vi "Get Data Refs.vi"(8 "error in (no error)":errorcluster, 9 "Access":T3, 10 "References":T1[](array[typedef]) format="%.0x", 11 "Item Ref in":T1 format="%.0x") -> (0 "error out":errorcluster, 2 "Data References":T2[](array[typedef]) format="%.0x", 3 "Device Ref out":T1 format="%.0x")   [LabVIEW 2021]
uses:
  <vilib>/NI VeriStand/Custom Device API/Data Access Type.ctl
  <vilib>/NI VeriStand/Custom Device API/Custom Device Item Ref.ctl
  <vilib>/NI VeriStand/Custom Device API/Data Reference.ctl
  <vilib>/NI VeriStand/Custom Device API/Custom Device API.lvlib
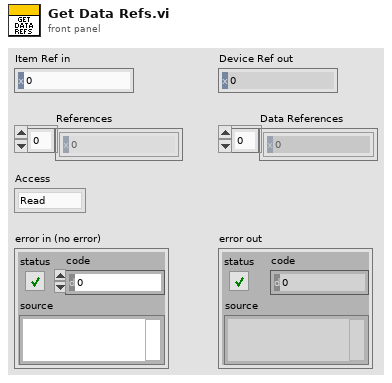
[diagram p1: front panel]
types:
  T1 = typedef "Custom Device API.lvlib/Custom Device Item Ref.ctl" = u64
  T2 = typedef "Custom Device API.lvlib/Data Reference.ctl" = i32
  T3 = typedef "Custom Device API.lvlib/Data Access Type.ctl" = enum16{"Read", "Write"}
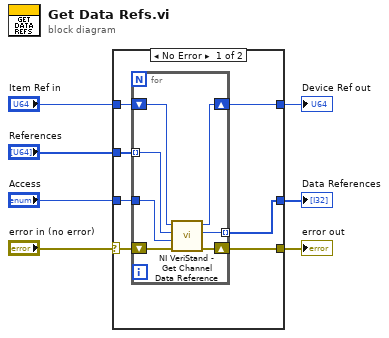
[diagram p0: block diagram]
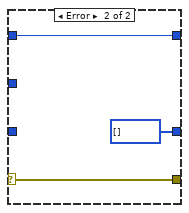
[diagram p2: hidden frame]
diagram:
  n1 = case shown="No Error" "error in (no error)" {
    selector: "error in (no error)" -> [w12 w22]
    tunnel: "Access" -> [w14 _]
    tunnel: [w13 w24] -> w6
    tunnel: [w11 w22] -> w4
    tunnel: "Item Ref in" -> [w10 w24]
    tunnel: "References" -> [w9 _]
    tunnel: [w8 T2[] []] -> w1
    frame No Error {
      n2 = for {
        shift-right: [w18] -> w13
        shift-left: w10 -> [w20]
        tunnel: w9 -> [w15] mode=indexing
        shift-right: [w19] -> w11
        shift-left: w12 -> [w21]
        tunnel: [w17] -> w8 mode=indexing
        tunnel: w14 -> [w16]
        n3 = call <vilib>:"NI VeriStand - Get Channel Data Reference.vi"("error in (no error)"=w21, "Access"=w16, "Channel Ref in"=w15, "Device Ref in"=w20) -> ("error out"=w19:errorcluster, "Channel Data Reference"=w17:T2, "Device Ref out"=w18:T1)  [unwired: 5 out]
      }
    }
    frame Error {
    }
  }
  "Device Ref out" <- w6
  "Data References" <- w1
  "error out" <- w4
